vi "PHY-2019-038.vi"() -> ()   [LabVIEW 2022 SP3]
panel:
  out "s":dbl
  in  "c":dbl
  in  "b":dbl
  in  "a":dbl
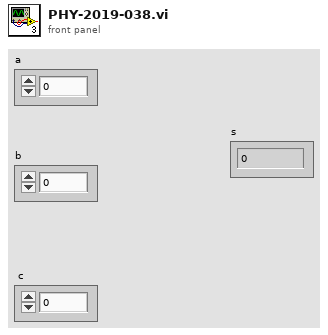
[diagram p1: front panel]
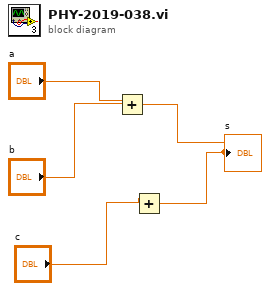
[diagram p0: block diagram]
diagram:
  n1 = Add(x="a", y="b") -> (x+y=w1:dbl)
  "s" <- w1
  n2 = Add(x="c", x+y=w1) -> ()  [unwired: 1 in]
